vi "ZLockReconnect.vi"(8 "error in (no error)":errorcluster, 11 "ZLock in":refnum<class "ZLock.lvclass">) -> (0 "error out":errorcluster, 3 "ZLock out":refnum<class "ZLock.lvclass">)   [LabVIEW 2012, in "ZLock.lvclass"]
uses:
  <userlib>/BIAS2/subvis/zlock/ZLock.lvclass
  <vilib>/addons/zeromq/socket_type.ctl
  <userlib>/BIAS2/subvis/zlock/ZLock.lvclass/ZLock.ctl
  <vilib>/addons/zeromq/zeromq.lvlib
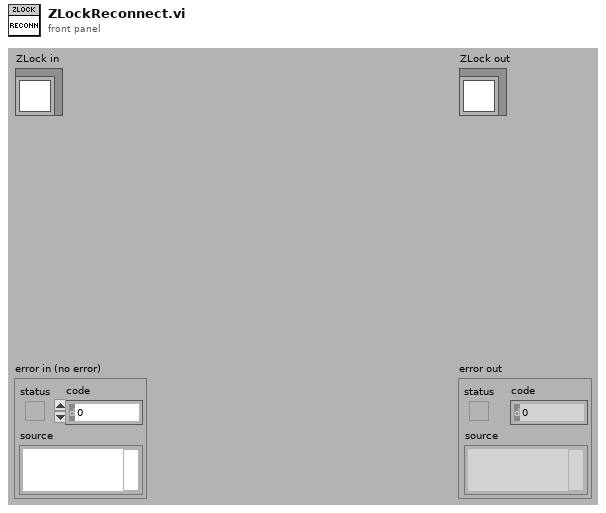
[diagram p1: front panel]
types:
  T1 = typedef "zeromq.lvlib/socket_type.ctl" = enum8{"ZMQ_PAIR", "ZMQ_PUB", "ZMQ_SUB", "ZMQ_REQ", "ZMQ_REP", "ZMQ_DEALER", "ZMQ_ROUTER", "ZMQ_PULL", "ZMQ_PUSH", "ZMQ_XPUB", "ZMQ_XSUB"}
  T2 = typedef "pointer.ctl" = u64
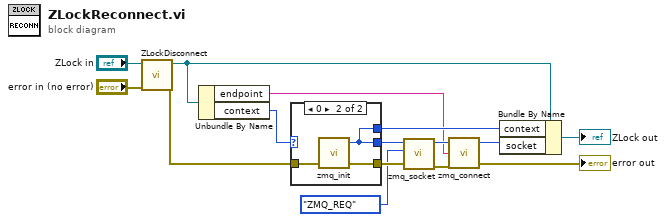
[diagram p0: block diagram]
diagram:
  n1 = call-dynamic "ZLockDisconnect.vi"("error in (no error)"="error in (no error)", "ZLock in"="ZLock in") -> ("error out"=w4:errorcluster, "ZLock out"=w1:refnum<class "ZLock.lvclass">)  [unwired: 8 in]
  n2 = Unbundle By Name(w1) -> ("endpoint"=w2:string, "context"=w3:T2)
  n3 = case shown="0" w3 {
    selector: w3 -> [w17 _]
    tunnel: [w17 w18] -> w9
    tunnel: [w16 w20] -> w11
    tunnel: w4 -> [w16 w19]
    tunnel: [_ w18] -> w5
    frame Default {
    }
    frame 0 {
      n4 = call <vilib>:"zmq_init.vi"("error in"=w19) -> ("error out"=w20:errorcluster, "context"=w18:T2)  [unwired: 3 in]
    }
  }
  n5 = call <vilib>:"zmq_socket.vi"("error in"=w11, "socket type"=socket_type."ZMQ_REQ", "ctx in"=w9) -> ("error out"=w10:errorcluster, "socket"=w7:T2)  [unwired: 3 in]
  n6 = call <vilib>:"zmq_connect.vi"("error in"=w10, "endpoint"=w2, "socket in"=w7) -> ("error out"=→"error out":errorcluster, "socket out"=w6:T2)  [unwired: 1 in]
  n7 = Bundle By Name(cluster=w1, "context"=w5, "socket"=w6) -> (→"ZLock out":refnum<class "ZLock.lvclass">)
